vi "AIT 1553 Parameter Page.vi"(8 "error in (no error)":errorcluster, 11 "Node Ptr":T3 format="%.0x") -> (0 "error out":errorcluster)   [LabVIEW 2011, in "AIT 1553 Custom Device.lvlib"]
uses:
  AIT 1553 Custom Device.lvlib
  <vilib>/NI Veristand/Custom Device API/Custom Device Item Ref.ctl
  Controls and Global/Start Bit.ctl
  Controls and Global/Number of Bits.ctl
  Controls/1553 Param.ctl
  Controls and Global/Global.vi
  <vilib>/NI Veristand/Custom Device API/Get Item Property (U32 Array).vi
  <vilib>/NI Veristand/Custom Device API/Get Item Property (Boolean).vi
  <vilib>/NI Veristand/Custom Device API/Get Item Property (U16).vi
  <vilib>/NI Veristand/Custom Device API/Get Item Property (Double).vi
  <vilib>/NI Veristand/Custom Device API/Get Item Property (I32).vi
  <vilib>/NI Veristand/Custom Device API/Set Item Property (U16).vi
  <vilib>/NI Veristand/Custom Device API/Set Item Property (I32).vi
  <vilib>/NI Veristand/Custom Device API/Set Item Property (Boolean).vi
  <vilib>/NI Veristand/Custom Device API/Set Item Property (Double).vi
  <vilib>/NI Veristand/Custom Device API/Custom Device API.lvlib
panel:
  in  "First Word":u16
  out "TriggerDValChange":bool
  in  "Scale Offset":dbl format="%#_6f"
  in  "Scale Factor":dbl format="%#_6f"
  in  "Signed?":bool
  out "Default Value":dbl
  in  "Number of Bits":T1=1 min=1 max=32
  in  "Start Bit":T2=1
  in  "Header":cluster{"Section Name":string}={"Section Name"="AIT 1553  Parameter"}
  in  "Description":string
  in  "Name":string
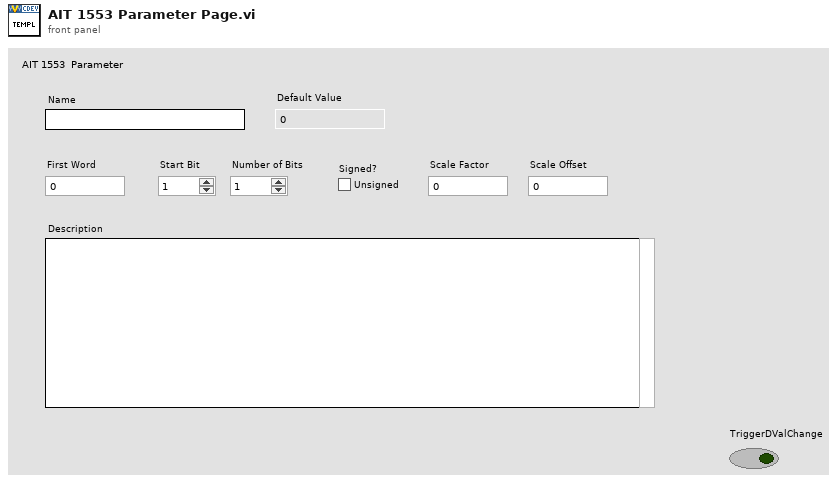
[diagram p1: front panel]
types:
  T1 = typedef "AIT 1553 Custom Device.lvlib/Number of Bits.ctl" = i32
  T2 = typedef "AIT 1553 Custom Device.lvlib/Start Bit.ctl" = i32
  T3 = typedef "Custom Device API.lvlib/Custom Device Item Ref.ctl" = u64
  T4 = typedef "Custom Device API.lvlib/Custom Device Item Info.ctl" = cluster{"Name":string, "Is Channel":bool, "GUID":string}
  T5 = typedef "Custom Device API.lvlib/Custom Device Channel.ctl" = cluster{"Type":T6, "Units":string, "Default Value":dbl, "Faultable":bool, "Scalable":bool}
  T6 = typedef "Custom Device API.lvlib/Custom Device Channel Type.ctl" = enum16{"Input", "Output"}
  T7 = typedef "AIT 1553 Custom Device.lvlib/1553 Param.ctl" = cluster{"name":string, "firstWord":i32, "startBit":i32, "numberBits":i32, "scaleFactor":dbl, "scaleOffset":dbl, "signed":bool}
  T8 = typedef "Custom Device API.lvlib/Custom Device Commands.ctl" = enum16{"Default", "Item renamed", "Shutdown", "Dynamic button pressed"}
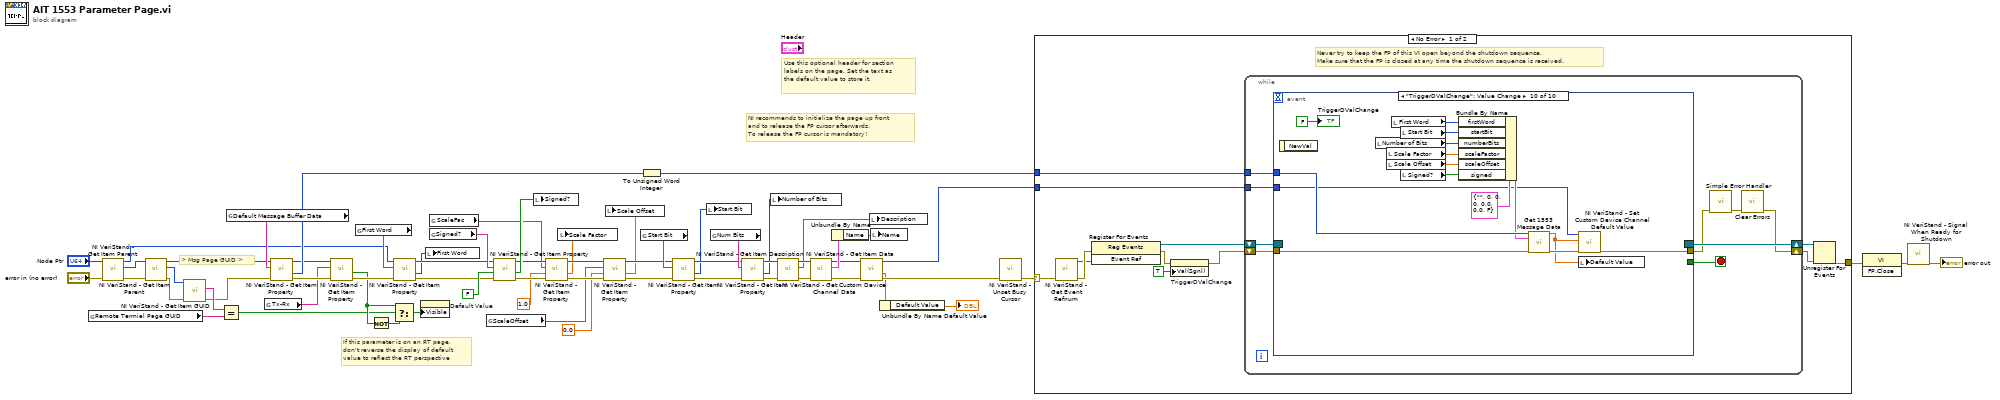
[diagram p0: block diagram]
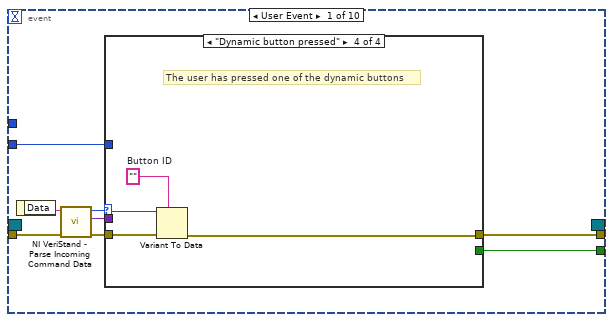
[diagram p2: hidden frame]
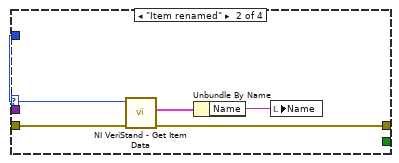
[diagram p4: hidden frame]
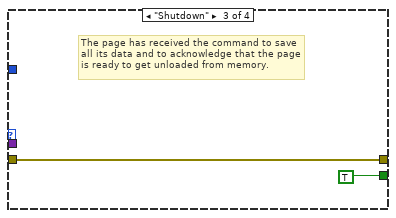
[diagram p5: hidden frame]
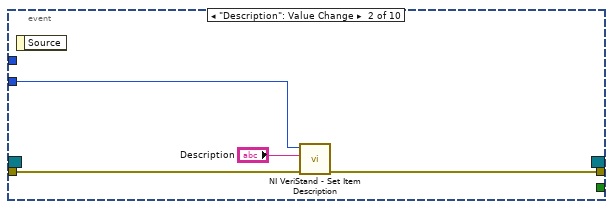
[diagram p6: hidden frame]
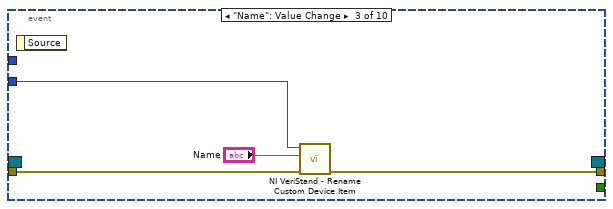
[diagram p7: hidden frame]
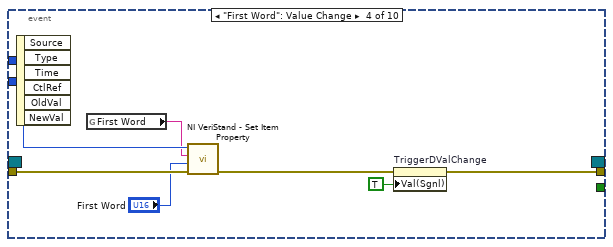
[diagram p8: hidden frame]
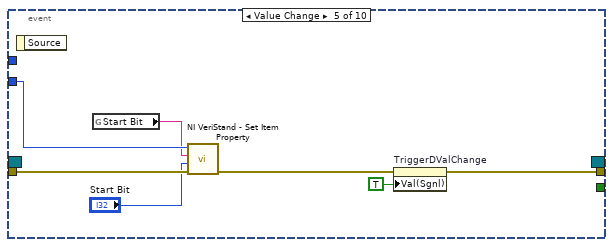
[diagram p9: hidden frame]
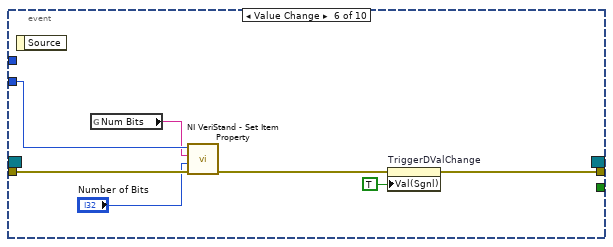
[diagram p10: hidden frame]
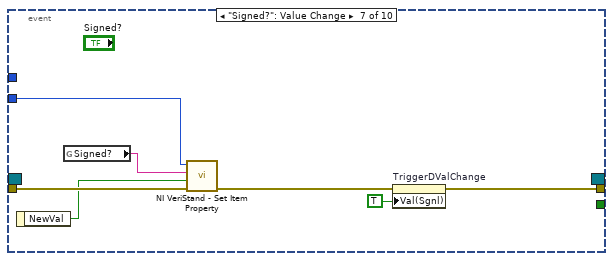
[diagram p11: hidden frame]
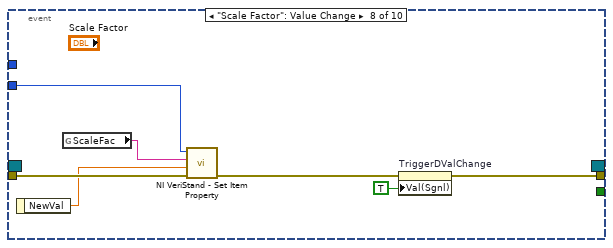
[diagram p12: hidden frame]
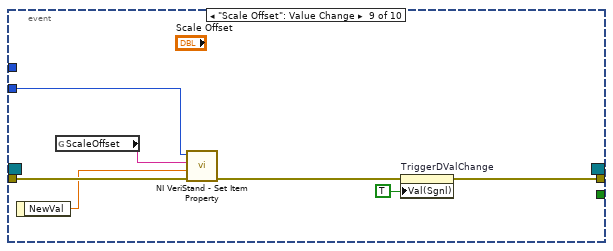
[diagram p13: hidden frame]
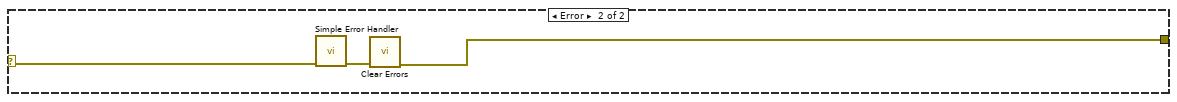
[diagram p14: hidden frame]
diagram:
  # "> Msg Page GUID >"
  # "If this parameter is on an RT page, \ndon't reverse the display of default\nvalue to reflect the RT perspective"
  # "Use this optional header for section labels on the page. Set the text as the default value to store it."
  # "NI recommends to initialize the page up front\nand to release the FP cursor afterwards.\nTo release the FP cursor is mandatory!"
  n1 = global read "Global.vi" "Remote Termial Page GUID"() -> (w5:string)
  n2 = call <vilib>:"NI VeriStand - Get Item Parent.vi"("error in (no error)"="error in (no error)", "Item Ref in"="Node Ptr") -> ("error out"=w12:errorcluster, "Parent Ref"=w13:T3, "Item Ref out"=w11:T3)  [unwired: 6 in, 1 out]
  n3 = call <vilib>:"NI VeriStand - Get Item Parent.vi"("error in (no error)"=w12, "Item Ref in"=w13) -> ("error out"=w8:errorcluster, "Parent Ref"=w9:T3, "Item Ref out"=w10:T3)  [unwired: 6 in, 1 out]
  n4 = call <vilib>:"NI VeriStand - Get Item GUID.vi"("error in (no error)"=w8, "Item Ref in"=w9) -> ("error out"=w6:errorcluster, "GUID"=w7:string)  [unwired: 7 in, 1 out]
  n5 = Equal?(x=w7, y=w5) -> (x = y?=w3:bool)
  n6 = global read "Global.vi" "Default Message Buffer Data"() -> (w41:string)
  n7 = global read "Global.vi" "Tx-Rx"() -> (w17:string)
  n8 = call-poly <vilib>:"NI VeriStand - Get Item Property.vi"("error in (no error)"=w6, "Property Name"=w41, "Item Ref in"=w10) -> ("error out"=w18:errorcluster, "Value"=w40:u32[], "Item Ref out"=w16:T3)  [unwired: 5 in, 1 out]
  n9 = call-poly <vilib>:"NI VeriStand - Get Item Property.vi"("error in (no error)"=w18, "Property Name"=w17, "Item Ref in"=w16) -> ("error out"=w15:errorcluster, "Value"=w4:bool)  [unwired: 5 in, 2 out]
  n10 = global read "Global.vi" "First Word"() -> (w20:string)
  n11 = Not(x=w4) -> (.not. x?=w2:bool)
  n12 = Select(t=w4, s=w3, f=w2) -> (s? t:f=w1:bool)
  n13 = call-poly <vilib>:"NI VeriStand - Get Item Property.vi"("error in (no error)"=w15, "Property Name"=w20, "Item Ref in"=w11) -> ("error out"=w22:errorcluster, "Value"=w19:u16, "Item Ref out"=w21:T3)  [unwired: 5 in, 1 out]
  n14 = property on="Default Value" class="DigNum (strict)"("Visible"=w1) -> ()  [unwired: 2 in, 2 out]
  n15 = local write "First Word"(w19) -> ()
  n16 = global read "Global.vi" "Signed?"() -> (w39:string)
  n17 = global read "Global.vi" "ScaleFac"() -> (w25:string)
  n18 = global read "Global.vi" "ScaleOffset"() -> (w29:string)
  n19 = call-poly <vilib>:"NI VeriStand - Get Item Property.vi"("error in (no error)"=w22, "Default Value"=FALSE, "Property Name"=w39, "Item Ref in"=w21) -> ("error out"=w36:errorcluster, "Value"=w37:bool, "Item Ref out"=w35:T3)  [unwired: 4 in, 1 out]
  n20 = local write "Signed?"(w37) -> ()
  n21 = call-poly <vilib>:"NI VeriStand - Get Item Property.vi"("error in (no error)"=w36, "Default Value"=1.0 ("Scale Factor"), "Property Name"=w25, "Item Ref in"=w35) -> ("error out"=w33:errorcluster, "Value"=w24:dbl, "Item Ref out"=w32:T3)  [unwired: 4 in, 1 out]
  n22 = local write "Scale Factor"(w24) -> ()
  n23 = call-poly <vilib>:"NI VeriStand - Get Item Property.vi"("error in (no error)"=w33, "Default Value"=0.0 ("Scale Factor"), "Property Name"=w29, "Item Ref in"=w32) -> ("error out"=w31:errorcluster, "Value"=w27:dbl, "Item Ref out"=w30:T3)  [unwired: 4 in, 1 out]
  n24 = local write "Scale Offset"(w27) -> ()
  n25 = To Unsigned Word Integer(number=w40) -> (unsigned 16bit integer=w26:u16[])
  n26 = global read "Global.vi" "Start Bit"() -> (w52:string)
  n27 = call-poly <vilib>:"NI VeriStand - Get Item Property.vi"("error in (no error)"=w31, "Property Name"=w52, "Item Ref in"=w30) -> ("error out"=w50:errorcluster, "Value"=w49:i32, "Item Ref out"=w51:T3)  [unwired: 5 in, 1 out]
  n28 = local write "Start Bit"(w49) -> ()
  n29 = global read "Global.vi" "Num Bits"() -> (w55:string)
  n30 = call-poly <vilib>:"NI VeriStand - Get Item Property.vi"("error in (no error)"=w50, "Property Name"=w55, "Item Ref in"=w51) -> ("error out"=w53:errorcluster, "Value"=w48:i32, "Item Ref out"=w54:T3)  [unwired: 5 in, 1 out]
  n31 = local write "Number of Bits"(w48) -> ()
  n32 = call <vilib>:"NI VeriStand - Get Item Description.vi"("error in (no error)"=w53, "Item Ref in"=w54) -> ("error out"=w58:errorcluster, "Description"=w59:string, "Item Ref out"=w60:T3)  [unwired: 7 out]
  n33 = call <vilib>:"NI VeriStand - Get Item Data.vi"("error in (no error)"=w58, "Item Ref in"=w60) -> ("error out"=w45:errorcluster, "Item Info"=w57:T4, "Item Ref out"=w44:T3)  [unwired: 7 out]
  n34 = Unbundle By Name(w57) -> ("Name"=w56:string)
  n35 = call <vilib>:"NI VeriStand - Get Custom Device Channel Data.vi"("error in (no error)"=w45, "Channel Ref in"=w44) -> ("error out"=w43:errorcluster, "Channel"=w42:T5, "Channel Ref out"=w14:T3)  [unwired: 4 in, 3 out]
  n36 = local write "Description"(w59) -> ()
  n37 = local write "Name"(w56) -> ()
  n38 = Unbundle By Name(w42) -> ("Default Value"=→"Default Value":dbl)
  n39 = call <vilib>:"NI VeriStand - Unset Busy Cursor.vi"("error in (no error)"=w43) -> ("error out"=w61:errorcluster)  [unwired: 10 out]
  n40 = case shown="No Error" w61 {
    selector: w61 -> [w69 w173]
    tunnel: [w73 w171] -> w64
    tunnel: w14 -> [w70 _]
    tunnel: w26 -> [w68 _]
    frame No Error {
      # "Never try to keep the FP of this VI open beyond the shutdown sequence.\nMake sure that the FP is closed at any time the shutdown sequence is received."
      n41 = call <vilib>:"NI VeriStand - Get Event Refnum.vi"("error in (no error)"=w69) -> ("error out"=w76:errorcluster, "Event Ref"=w72:refnum<user-event>)  [unwired: 9 out]
      n42 = register-events(error in=w76, w72) -> (reference out=w71:refnum<event-registration>, error out=w66:errorcluster)  [unwired: 1 in]
      n43 = property on="TriggerDValChange" class="Bool (strict)"(error in=w66, "Val(Sgnl)"=TRUE ("Value (Signaling)")) -> (error out=w65:errorcluster)  [unwired: 1 in, 1 out]
      n44 = while {
        tunnel: w70 -> [w81]
        shift-right: [w78] -> w74
        shift-left: w65 -> [w84]
        shift-right: [w85] -> w75
        shift-left: w71 -> [w83]
        tunnel: w68 -> [w77]
        stop <- w82 stop-if-true
        n45 = event shown="[9] \"TriggerDValChange\": Value Change" {
          selector: w83 -> [_ _ _ _ _ _ _ _ _ _]
          dyn-events: [_ _ _ _ _ _ _ _ _ _] -> w85
          timeout: _ -> [_ _ _ _ _ _ _ _ _ _]
          tunnel: w84 -> [w93 w108 w112 w120 w127 w134 w141 w148 w155 w159]
          tunnel: [w89 _ _ _ _ _ _ _ _ _] -> w82
          tunnel: [w88 w107 w111 w116 w123 w128 w135 w142 w149 w170] -> w80
          tunnel: w81 -> [w87 w109 w113 w119 w126 w133 w140 w147 w154 w157]
          tunnel: w77 -> [_ _ _ _ _ _ _ _ _ w168]
          event User Event {
            n46 = event-data() -> ("Data"=w92:string)  [unwired: 1 out]
            n47 = call <vilib>:"NI VeriStand - Parse Incoming Command Data.vi"("error in (no error)"=w93, "Incoming data"=w92) -> ("error out"=w91:errorcluster, "Outgoing data"=w86:variant, "Action"=w90:T8)  [unwired: 7 out]
            n48 = case shown="\"Dynamic button pressed\"" w90 {
              tunnel: w91 -> [w94 w99 w100 w105]
              tunnel: [_ _ TRUE _] -> w89
              tunnel: [w94 w96 w100 w102] -> w88
              tunnel: w87 -> [_ w98 _ _]
              tunnel: w86 -> [_ _ _ w104]
              frame "Default", Default {
              }
              frame "Item renamed" {
                n49 = call <vilib>:"NI VeriStand - Get Item Data.vi"("error in (no error)"=w99, "Item Ref in"=w98) -> ("error out"=w96:errorcluster, "Item Info"=w97:T4)  [unwired: 8 out]
                n50 = Unbundle By Name(w97) -> ("Name"=w95:string)
                n51 = local write "Name"(w95) -> ()
              }
              frame "Shutdown" {
                # "The page has received the command to save all its data and to acknowledge that the page is ready to get unloaded from memory."
              }
              frame "Dynamic button pressed" {
                w103 = ""  # Button ID
                # "The user has pressed one of the dynamic buttons"
                n52 = Variant To Data(error in=w105, type=w103, Variant=w104) -> (error out=w102:errorcluster)  [unwired: 1 out]
              }
            }
          }
          event "Description": Value Change {
            n53 = event-data() -> ()  [unwired: 2 out]
            n54 = call <vilib>:"NI VeriStand - Set Item Description.vi"("error in (no error)"=w108, "Description"="Description", "Item Ref in"=w109) -> ("error out"=w107:errorcluster)  [unwired: 8 out]
          }
          event "Name": Value Change {
            n55 = event-data() -> ()  [unwired: 2 out]
            n56 = call <vilib>:"NI VeriStand - Rename Custom Device Item.vi"("error in (no error)"=w112, "New Name"="Name", "Item Ref in"=w113) -> ("error out"=w111:errorcluster)  [unwired: 6 in, 2 out]
          }
          event "First Word": Value Change {
            n57 = event-data() -> ()  [unwired: 7 out]
            n58 = global read "Global.vi" "First Word"() -> (w118:string)
            n59 = call-poly <vilib>:"NI VeriStand - Set Item Property.vi"("error in (no error)"=w120, "Value"="First Word", "Property Name"=w118, "Item Ref in"=w119) -> ("error out"=w117:errorcluster)  [unwired: 5 in, 2 out]
            n60 = property on="TriggerDValChange" class="Bool (strict)"(error in=w117, "Val(Sgnl)"=TRUE ("Value (Signaling)")) -> (error out=w116:errorcluster)  [unwired: 1 in, 1 out]
          }
          event Value Change {
            n61 = event-data() -> ()  [unwired: 2 out]
            n62 = global read "Global.vi" "Start Bit"() -> (w125:string)
            n63 = call-poly <vilib>:"NI VeriStand - Set Item Property.vi"("error in (no error)"=w127, "Value"="Start Bit", "Property Name"=w125, "Item Ref in"=w126) -> ("error out"=w124:errorcluster)  [unwired: 5 in, 2 out]
            n64 = property on="TriggerDValChange" class="Bool (strict)"(error in=w124, "Val(Sgnl)"=TRUE ("Value (Signaling)")) -> (error out=w123:errorcluster)  [unwired: 1 in, 1 out]
          }
          event Value Change {
            n65 = event-data() -> ()  [unwired: 2 out]
            n66 = global read "Global.vi" "Num Bits"() -> (w132:string)
            n67 = call-poly <vilib>:"NI VeriStand - Set Item Property.vi"("error in (no error)"=w134, "Value"="Number of Bits", "Property Name"=w132, "Item Ref in"=w133) -> ("error out"=w129:errorcluster)  [unwired: 5 in, 2 out]
            n68 = property on="TriggerDValChange" class="Bool (strict)"(error in=w129, "Val(Sgnl)"=TRUE ("Value (Signaling)")) -> (error out=w128:errorcluster)  [unwired: 1 in, 1 out]
          }
          event "Signed?": Value Change {
            n69 = event-data() -> ("NewVal"=w138:bool)  [unwired: 1 out]
            n70 = global read "Global.vi" "Signed?"() -> (w139:string)
            n71 = call-poly <vilib>:"NI VeriStand - Set Item Property.vi"("error in (no error)"=w141, "Value"=w138, "Property Name"=w139, "Item Ref in"=w140) -> ("error out"=w136:errorcluster)  [unwired: 5 in, 2 out]
            n72 = property on="TriggerDValChange" class="Bool (strict)"(error in=w136, "Val(Sgnl)"=TRUE ("Value (Signaling)")) -> (error out=w135:errorcluster)  [unwired: 1 in, 1 out]
          }
          event "Scale Factor": Value Change {
            n73 = event-data() -> ("NewVal"=w145:dbl)  [unwired: 1 out]
            n74 = global read "Global.vi" "ScaleFac"() -> (w146:string)
            n75 = call-poly <vilib>:"NI VeriStand - Set Item Property.vi"("error in (no error)"=w148, "Value"=w145, "Property Name"=w146, "Item Ref in"=w147) -> ("error out"=w143:errorcluster)  [unwired: 5 in, 2 out]
            n76 = property on="TriggerDValChange" class="Bool (strict)"(error in=w143, "Val(Sgnl)"=TRUE ("Value (Signaling)")) -> (error out=w142:errorcluster)  [unwired: 1 in, 1 out]
          }
          event "Scale Offset": Value Change {
            n77 = event-data() -> ("NewVal"=w152:dbl)  [unwired: 1 out]
            n78 = global read "Global.vi" "ScaleOffset"() -> (w153:string)
            n79 = call-poly <vilib>:"NI VeriStand - Set Item Property.vi"("error in (no error)"=w155, "Value"=w152, "Property Name"=w153, "Item Ref in"=w154) -> ("error out"=w150:errorcluster)  [unwired: 5 in, 2 out]
            n80 = property on="TriggerDValChange" class="Bool (strict)"(error in=w150, "Val(Sgnl)"=TRUE ("Value (Signaling)")) -> (error out=w149:errorcluster)  [unwired: 1 in, 1 out]
          }
          event "TriggerDValChange": Value Change {
            n81 = event-data() -> ()  [unwired: 2 out]
            n82 = local read "Number of Bits"() -> (w165:T1)
            n83 = local read "Scale Factor"() -> (w164:dbl)
            n84 = local read "Scale Offset"() -> (w163:dbl)
            n85 = local read "First Word"() -> (w161:u16)
            n86 = local read "Start Bit"() -> (w166:T2)
            n87 = local read "Signed?"() -> (w160:bool)
            n88 = Bundle By Name(cluster=T7 {"name"="", "firstWord"=0, "startBit"=0, "numberBits"=0, "scaleFactor"=0.0, "scaleOffset"=0.0, "signed"=FALSE} ("1553 Parameter"), "firstWord"=w161, "startBit"=w166, "numberBits"=w165, "scaleFactor"=w164, "scaleOffset"=w163, "signed"=w160) -> (w162:T7)
            n89 = call "Get 1553 Message Data.vi"("MSG DATA"=w168, "1553 Parameter"=w162, "error in (no error)"=w159) -> ("Value"=w156:dbl, "error out"=w158:errorcluster)  [unwired: 11 in]
            n90 = call <vilib>:"NI VeriStand - Set Custom Device Channel Default Value.vi"("error in (no error)"=w158, "Default Value"=w156, "Channel Ref in"=w157) -> ("error out"=w170:errorcluster)  [unwired: 7 in, 1 out]
            n91 = local write "Default Value"(w156) -> ()
            "TriggerDValChange" <- FALSE
          }
        }
        n92 = call <vilib>:"Simple Error Handler.vi"("error in (no error)"=w80) -> ("error out"=w79:errorcluster)  [unwired: 1 in, 7 out]
        n93 = call <vilib>:"Clear Errors.vi"("error in (no error)"=w79) -> ("error out"=w78:errorcluster)  [unwired: 6 out]
      }
      n94 = Unregister For Events(event registration refnum=w75, error in=w74) -> (error out=w73:errorcluster)
    }
    frame Error {
      n95 = call <vilib>:"Simple Error Handler.vi"("error in (no error)"=w173) -> ("error out"=w172:errorcluster)  [unwired: 1 in, 7 out]
      n96 = call <vilib>:"Clear Errors.vi"("error in (no error)"=w172) -> ("error out"=w171:errorcluster)  [unwired: 6 out]
    }
  }
  n97 = invoke class="VI" method="FP.Close"(error in=w64) -> (error out=w63:errorcluster)  [unwired: 2 in, 2 out]
  n98 = call <vilib>:"NI VeriStand - Signal When Ready for Shutdown.vi"("error in (no error)"=w63) -> ("error out"=→"error out":errorcluster)  [unwired: 10 out]
